vi "Write Max File Size.vi"(8 "error in (no error)":errorcluster, 10 "Max File Size":i32, 11 "EHVIT Logger in":refnum<class "Logger.lvclass">) -> (0 "error out":errorcluster, 3 "EHVIT Logger out":refnum<class "Logger.lvclass">)   [LabVIEW 2017, in "Logger.lvlib" / "Logger.lvclass"]
uses:
  Logger.lvclass
  Logger.lvclass/Logger.ctl
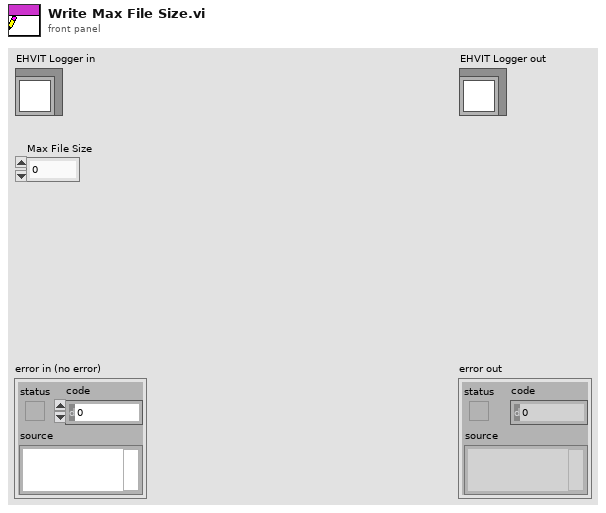
[diagram p1: front panel]
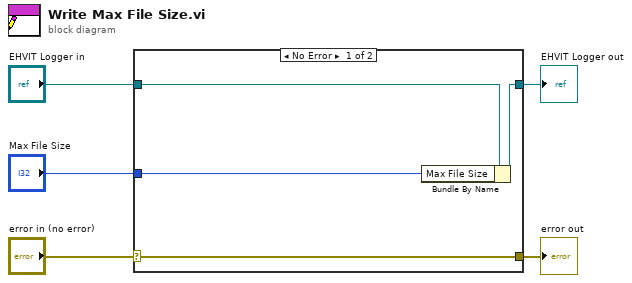
[diagram p0: block diagram]
diagram:
  n1 = case shown="No Error" "error in (no error)" {
    selector: "error in (no error)" -> [w9 w10]
    tunnel: [w9 w10] -> w4
    tunnel: [w7 w11] -> w2
    tunnel: "EHVIT Logger in" -> [w8 w11]
    tunnel: "Max File Size" -> [w6 _]
    frame No Error {
      n2 = Bundle By Name(cluster=w8, "Max File Size"=w6) -> (w7:refnum<class "Logger.lvclass">)
    }
    frame Error {
    }
  }
  "error out" <- w4
  "EHVIT Logger out" <- w2
